vi "addReading.vi"(8 "error in (no error)":errorcluster, 10 "reading":T1, 11 "ElectrometerController in":refnum<class "ElectrometerController.lvclass">) -> (0 "error out":errorcluster, 3 "ElectrometerController out":refnum<class "ElectrometerController.lvclass">)   [LabVIEW 2016, in "ElectrometerController.lvclass"]
uses:
  ElectrometerController.lvclass
  ts_electrometeruserevents/Typedefs/Reading.ctl
  ElectrometerController.lvclass/ElectrometerController.ctl
  ts_electrometeruserevents/Typedefs/ElectrometerTypedefs.lvlib
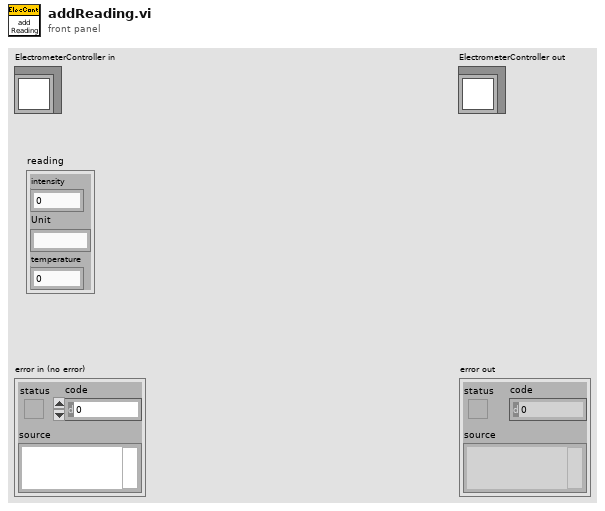
[diagram p1: front panel]
types:
  T1 = typedef "ElectrometerTypedefs.lvlib/Reading.ctl" = cluster{"intensity":dbl, "Unit":string, "temperature":dbl}
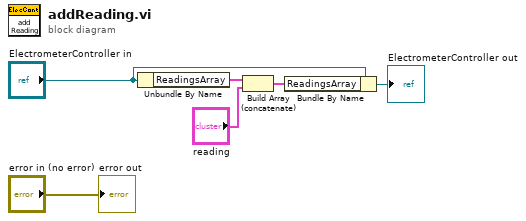
[diagram p0: block diagram]
diagram:
  n1 = Unbundle By Name("ElectrometerController in") -> ("ReadingsArray"=w3:T1[])
  n2 = Build Array (concatenate)(w3, "reading") -> (w1:T1[])
  n3 = Bundle By Name(cluster="ElectrometerController in", "ReadingsArray"=w1) -> (→"ElectrometerController out":refnum<class "ElectrometerController.lvclass">)
  "error out" <- "error in (no error)"
